vi "WrapPhase180.vi"(2 "dPhi":dbl, 3 "VDUT/VRef":dbl) -> (0 "Wrapped\nPhase\nDifference\n(-180,180]":dbl, 1 "Gain (dB)":dbl)   [LabVIEW 2026]
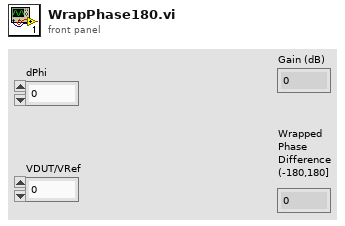
[diagram p1: front panel]
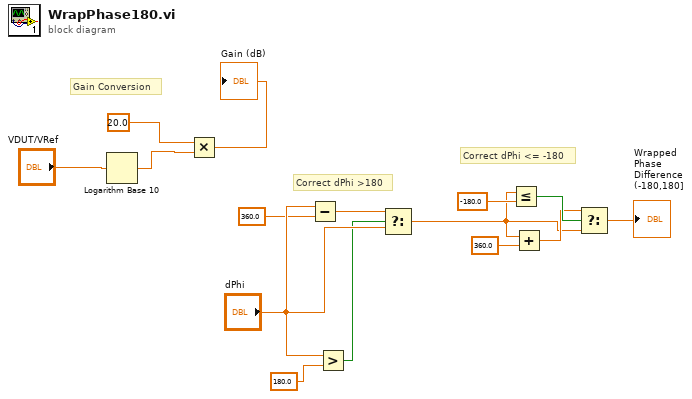
[diagram p0: block diagram]
diagram:
  # "Correct dPhi <= -180"
  # "Correct dPhi >180"
  # "Gain Conversion"
  n1 = Logarithm Base 10(1:"VDUT/VRef") -> (0:w7:dbl)
  n2 = Multiply(x=20.0, y=w7) -> (x*y=→"Gain (dB)":dbl)
  n3 = Subtract(x="dPhi", y=360.0) -> (x-y=w12:dbl)
  n4 = Greater?(x="dPhi", y=180.0) -> (0:w11:bool)
  n5 = Select(t=w12, s=w11, f="dPhi") -> (s? t:f=w2:dbl)
  n6 = Less Or Equal?(x=w2, y=-180.0) -> (x <= y?=w4:bool)
  n7 = Add(x=w2, y=360.0) -> (x+y=w3:dbl)
  n8 = Select(t=w3, s=w4, f=w2) -> (s? t:f=→"Wrapped\nPhase\nDifference\n(-180,180]":dbl)
